vi "command movr.vi"(8 "error in (no error)":errorcluster, 9 "uDeltaPosition":i32, 10 "DeltaPosition":i32, 11 "id":i32) -> (0 "error out":errorcluster, 3 "function return":i32)   [LabVIEW 2012, in "libximc.lvlib"]
doc: "result_t XIMC_API command_movr (device_t id, int DeltaPosition, int uDeltaPosition);"
uses:
  libximc.lvlib
  libximc.dll
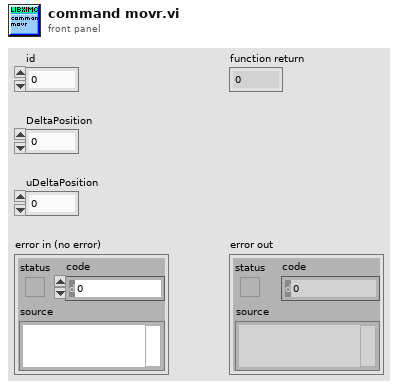
[diagram p1: front panel]
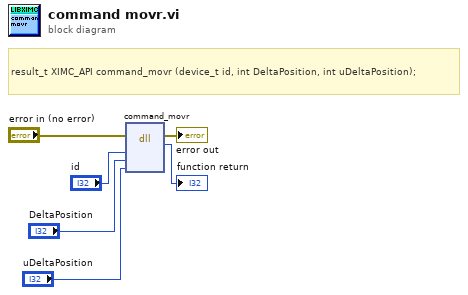
[diagram p0: block diagram]
diagram:
  # "result_t XIMC_API command_movr (device_t id, int DeltaPosition, int uDeltaPosition);"
  n1 = dll-call lib="C:/Users/Stepan/Downloads/labview_2.9.11_testgen_thread/libximc.*" fn="command_movr"(error in="error in (no error)", "id"="id", "DeltaPosition"="DeltaPosition", "uDeltaPosition"="uDeltaPosition") -> (error out=→"error out":errorcluster, →"function return":i32)  [unwired: 5 in, 1 out]
